vi "Fuel Flow to RPM.vi"(11 "Fuel Pump Value 1":i32) -> (3 "RPM":dbl=44000.0 min=44000.0 max=135000.0)   [LabVIEW 2017]
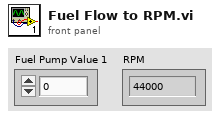
[diagram p1: front panel]
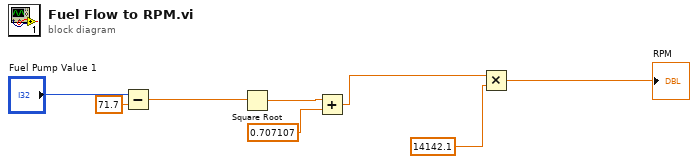
[diagram p0: block diagram]
diagram:
  n1 = Subtract(x="Fuel Pump Value 1", y=71.7) -> (x-y=w4:dbl)
  n2 = Square Root(x=w4) -> (sqrt(x)=w3:dbl)
  n3 = Add(x=w3, y=0.707107) -> (x+y=w1:dbl)
  n4 = Multiply(x=w1, y=14142.1) -> (x*y=→"RPM":dbl)
